vi "Write Low Time.vi"(8 "error in (no error)":errorcluster, 10 "Low Time":u32, 11 "Servo Switch in":refnum<class "Servo Switch.lvclass">) -> (0 "error out":errorcluster, 3 "Servo Switch out":refnum<class "Servo Switch.lvclass">)   [LabVIEW 2019, in "Servo Switch.lvclass"]
uses:
  Servo Switch.lvclass
  Servo Switch.lvclass/Servo Switch.ctl
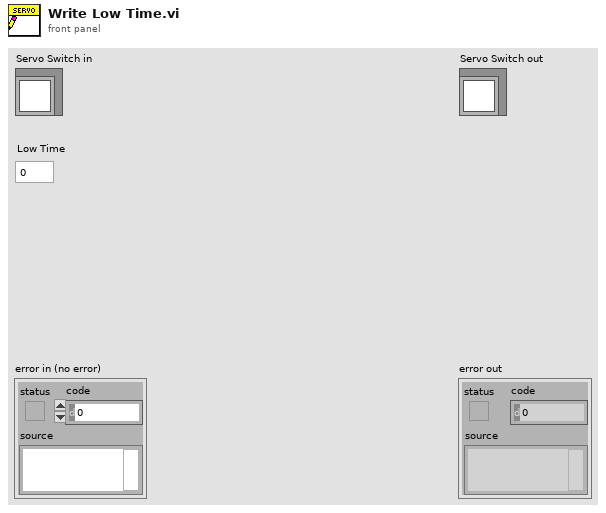
[diagram p1: front panel]
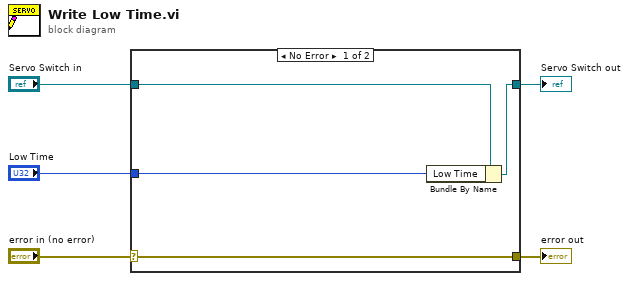
[diagram p0: block diagram]
diagram:
  n1 = case shown="No Error" "error in (no error)" {
    selector: "error in (no error)" -> [w9 w10]
    tunnel: [w9 w10] -> w4
    tunnel: [w7 w11] -> w2
    tunnel: "Servo Switch in" -> [w8 w11]
    tunnel: "Low Time" -> [w6 _]
    frame No Error {
      n2 = Bundle By Name(cluster=w8, "Low Time"=w6) -> (w7:refnum<class "Servo Switch.lvclass">)
    }
    frame Error {
    }
  }
  "error out" <- w4
  "Servo Switch out" <- w2
